vi "Simple Track.vi"(10 "time delay":dbl) -> ()   [LabVIEW 2011]
uses:
  Robot Global Data.vi
  System Set Points and States.vi
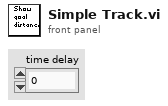
[diagram p1: front panel]
types:
  T1 = cluster{"Position":cluster{"X":dbl, "Y":dbl}, "Distance (ft)":dbl}[]
  T2 = cluster{"Target Info[0]":cluster{"Position":cluster{"X":dbl, "Y":dbl}, "Distance (ft)":dbl}, "Target Info[1]":cluster{"Position":cluster{"X":dbl, "Y":dbl}, "Distance (ft)":dbl}, "Target Info[2]":cluster{"Position":cluster{"X":dbl, "Y":dbl}, "Distance (ft)":dbl}, "Target Info[3]":cluster{"Position":cluster{"X":dbl, "Y":dbl}, "Distance (ft)":dbl}, "Target Info[4]":cluster{"Position":cluster{"X":dbl, "Y":dbl}, "Distance (ft)":dbl}, "Target Info[5]":cluster{"Position":cluster{"X":dbl, "Y":dbl}, "Distance (ft)":dbl}, "Target Info[6]":cluster{"Position":cluster{"X":dbl, "Y":dbl}, "Distance (ft)":dbl}, "Target Info[7]":cluster{"Position":cluster{"X":dbl, "Y":dbl}, "Distance (ft)":dbl}, "Target Info[8]":cluster{"Position":cluster{"X":dbl, "Y":dbl}, "Distance (ft)":dbl}}
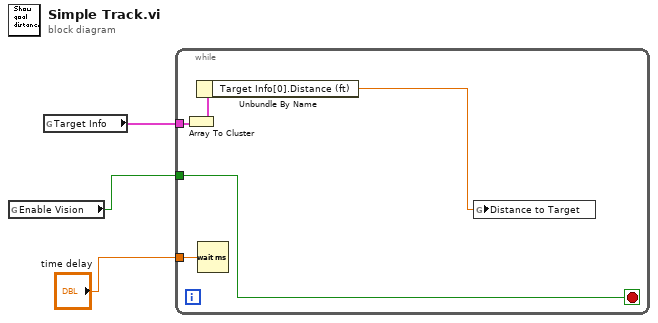
[diagram p0: block diagram]
diagram:
  n1 = global read "Robot Global Data.vi" "Enable Vision"() -> (w2:bool)
  n2 = global read "Robot Global Data.vi" "Target Info"() -> (w3:T1)
  n3 = while {
    tunnel: w3 -> [w8]
    tunnel: w2 -> [w5]
    tunnel: "time delay" -> [w4]
    stop <- w5 stop-if-true
    n4 = Array To Cluster(array=w8) -> (cluster=w7:T2)
    n5 = Unbundle By Name(w7) -> ("Target Info[0].Distance (ft)"=w6:dbl)
    n6 = Wait (ms)(milliseconds to wait=w4) -> ()  [unwired: 1 out]
    n7 = global write "System Set Points and States.vi" "Distance to Target"(w6) -> ()
  }
